vi "FLL Tournament Display Widescreen.vi"() -> ()   [LabVIEW 2013]
uses:
  Team_List_Ctrl.ctl
  Team_Scores_And_Rankings_Array_Ctrl.ctl
  Round_And_Score_Ctrl.ctl
  Timer_Details_Ctrl.ctl
  Sound Info.ctl
  <vilib>/sound2/lvsound2.llb/Sound Data Format.ctl
  <vilib>/sound2/lvsound2.llb/Sampling Mode.ctl
  SponsorImageFreqArray.ctl
  <vilib>/picture/picture.llb/imagedata.ctl
  <vilib>/sound2/lvsound2.llb/Sound Output Set Volume (Single).vi
  <vilib>/sound2/lvsound2.llb/Sound Output Write (DBL).vi
  <vilib>/httpClient/LabVIEWHTTPClient.lvlib
panel:
  out "TimerIP":string
  in  "Hurry-Up Sound Volume":dbl(slide)=88.46153846153847 scale=0.0..100.0
  in  "Pre-Match Coundown Sound Volume":dbl(slide)=88.46153846153847 scale=0.0..100.0
  in  "Uh-Oh Sound Volume":dbl(slide)=88.46153846153847 scale=0.0..100.0
  in  "Stop Sound Volume":dbl(slide)=100.0 scale=0.0..100.0
  in  "Start Sound Volume":dbl(slide)=100.0 scale=0.0..100.0
  out "Sound Cluster 2":T1={"Start"={"total number of samples/ch"=31680, "sound format"={"sample rate (S/s)"=11025.0, "number of channels"=1, "bits per sample"=16}, "data"=[{"t0"=timestamp(0 s since 1904-01-01), "dt"=9.070294784580499e-05, "Y"=array[31680 elements]}], "Volume"=100.0}, "Stop"={"total number of samples/ch"=27648, "sound format"={"sample rate (S/s)"=11025.0, "number of channels"=1, "bits per sample"=16}, "data"=[{"t0"=timestamp(0 s since 1904-01-01), "dt"=9.070294784580499e-05, "Y"=array[27648 elements]}], "Volume"=100.0}, "Uh-Oh"={"total number of samples/ch"=29952, "sound format"={"sample rate (S/s)"=11025.0, "number of channels"=1, "bits per sample"=16}, "data"=[{"t0"=timestamp(0 s since 1904-01-01), "dt"=9.070294784580499e-05, "Y"=array[29952 elements]}], "Volume"=88.46153846153847}, "PreMatch"={"total number of samples/ch"=225792, "sound format"={"sample rate (S/s)"=44100.0, "number of channels"=2, "bits per sample"=16}, "data"=[{"t0"=timestamp(0 s since 1904-01-01), "dt"=2.2675736961451248e-05, "Y"=array[225792 elements]}, {"t0"=timestamp(0 s since 1904-01-01), "dt"=2.2675736961451248e-05, "Y"=array[225792 elements]}], "Volume"=75.38461538461539}, "Hurry-Up"={"total number of samples/ch"=0, "sound format"={"sample rate (S/s)"=0.0, "number of channels"=0, "bits per sample"=0}, "data"=[], "Volume"=0.0}}
  in  "stop":bool
  in  "Sound To Play":T3(ring)
  out "Primary Sound Array":dbl[](array[numeric])
  out "PrePrimary Sound Array":dbl[](array[numeric])
  out "Secondary (s)":dbl
  out "Primary (s)":dbl
  out "Pre-Primary (s)":dbl
  out "Master Volume":dbl
  out "Sound Cluster":T1={"Start"={"total number of samples/ch"=31680, "sound format"={"sample rate (S/s)"=11025.0, "number of channels"=1, "bits per sample"=16}, "data"=[{"t0"=timestamp(0 s since 1904-01-01), "dt"=9.070294784580499e-05, "Y"=array[31680 elements]}], "Volume"=100.0}, "Stop"={"total number of samples/ch"=27648, "sound format"={"sample rate (S/s)"=11025.0, "number of channels"=1, "bits per sample"=16}, "data"=[{"t0"=timestamp(0 s since 1904-01-01), "dt"=9.070294784580499e-05, "Y"=array[27648 elements]}], "Volume"=100.0}, "Uh-Oh"={"total number of samples/ch"=29952, "sound format"={"sample rate (S/s)"=11025.0, "number of channels"=1, "bits per sample"=16}, "data"=[{"t0"=timestamp(0 s since 1904-01-01), "dt"=9.070294784580499e-05, "Y"=array[29952 elements]}], "Volume"=88.46153846153847}, "PreMatch"={"total number of samples/ch"=225792, "sound format"={"sample rate (S/s)"=44100.0, "number of channels"=2, "bits per sample"=16}, "data"=[{"t0"=timestamp(0 s since 1904-01-01), "dt"=2.2675736961451248e-05, "Y"=array[225792 elements]}, {"t0"=timestamp(0 s since 1904-01-01), "dt"=2.2675736961451248e-05, "Y"=array[225792 elements]}], "Volume"=75.38461538461539}, "Hurry-Up"={"total number of samples/ch"=0, "sound format"={"sample rate (S/s)"=0.0, "number of channels"=0, "bits per sample"=0}, "data"=[], "Volume"=0.0}}
  out "EnableSounds":bool
  out "Score Behavior":T4(ring)
  out "SFA":string[][](array[string])
  out "NumRoundsToShow":string
  out "Cancelled?":bool
  out "IP Address / Port":string
  in  "Scores Tab":enum32{"3 Rounds", "4 Rounds"}(tab)
  in  "Scores Box":i32[](listbox)
  in  "Scores Box 2":i32(listbox)=3
  in  "Top Tab":enum32{"Page 1"}(tab)
  out "Main Logo Image":picture
  out "Powered By LabVIEW":picture
  out "FIRST LEGO League":picture
  out "Match Indicator":string
  out "Tournament Title String":string="2013 FIRST LEGO League Nature's Fury"
  out "TIMER":string="2 : 3 0"
  out "Top Sponsor Image":picture
  out "Mid Sponsor Image":picture
  out "Bottom Sponsor Image":picture
  out "Timer Properties":T5
  out "Consolidated Scores and Rankings":T7(array[cluster])
  out "Reported Scores and Rankings":T8
  out "Full Team List":T9[](array[typedef])
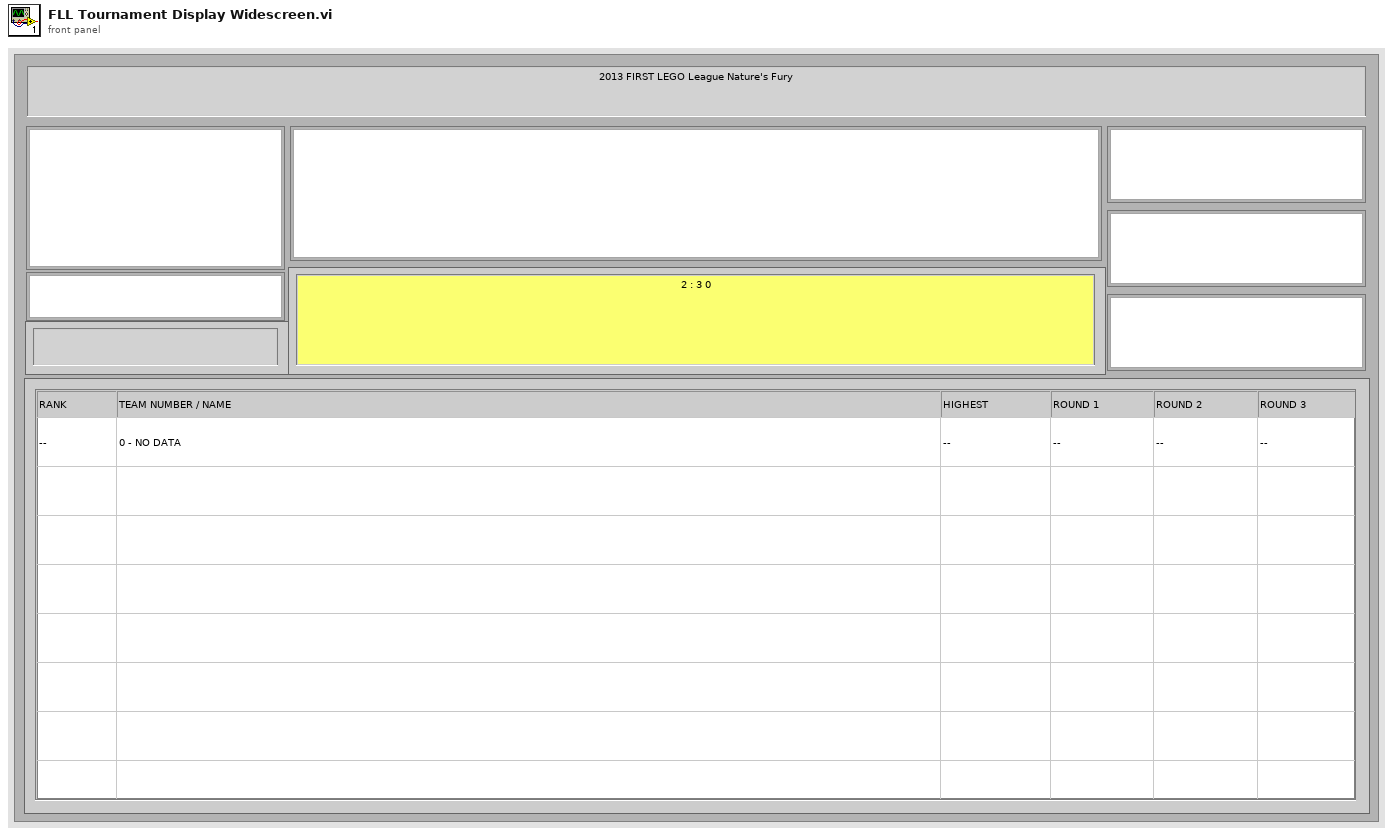
[diagram p1: front panel]
types:
  T1 = typedef "Sound Info.ctl" = cluster{"Start":cluster{"total number of samples/ch":u32, "sound format":T2, "data":waveform(dbl)[], "Volume":dbl}, "Stop":cluster{"total number of samples/ch":u32, "sound format":T2, "data":waveform(dbl)[], "Volume":dbl}, "Uh-Oh":cluster{"total number of samples/ch":u32, "sound format":T2, "data":waveform(dbl)[], "Volume":dbl}, "PreMatch":cluster{"total number of samples/ch":u32, "sound format":T2, "data":waveform(dbl)[], "Volume":dbl}, "Hurry-Up":cluster{"total number of samples/ch":u32, "sound format":T2, "data":waveform(dbl)[], "Volume":dbl}}
  T2 = typedef "Sound Data Format.ctl" = cluster{"sample rate (S/s)":dbl, "number of channels":i32, "bits per sample":i32}
  T3 = enum16{"None", "Start", "Stop", "Uh-Oh", "Prematch", "Hurry-Up"}
  T4 = enum16{"Show Negative Scores as ZERO", "Show Negative Scores"}
  T5 = typedef "Timer_Details_Ctrl.ctl" = cluster{"TimeRemaining":string, "MatchPhase":string, "CurrentMatch":string, "Timer_Running":string, "Seconds":string, "LastSound":string}
  T6 = typedef "Round_And_Score_Ctrl.ctl" = cluster{"Score":string, "Round Number":string}
  T7 = cluster{"Rank":string, "Team Number":string, "Team Name":string, "Highest Score":string, "Scores":T6[]}[]
  T8 = typedef "Team_Scores_And_Rankings_Array_Ctrl.ctl" = cluster{"Rank":string, "Team Number":string, "Team Name":string, "Highest Score":string, "Scores":T6[]}[]
  T9 = typedef "Team_List_Ctrl.ctl" = cluster{"Team Name":string, "Team Number":string}
  T10 = enum32{"Invalid", "Standard", "Closed", "Hidden", "Minimized", "Maximized"}
  T11 = cluster{"Master Volume":dbl, "Pre-Primary (s)":dbl, "Primary (s)":dbl, "Secondary (s)":dbl, "Start Sound Path":path, "Stop Sound Path":path, "Uh-Oh Sound Path":path, "Pre-Match Countdown Sound":path, "Hurry Up Sound":path, "Start Sound Volume":dbl, "Stop Sound Volume":dbl, "Uh-Oh Sound Volume":dbl, "Pre-Match Coundown Sound Volume":dbl, "Hurry Up Sound Volume":dbl}
  T12 = typedef "SponsorImageFreqArray.ctl" = cluster{"Cluster":cluster{"Array":T13[], "Frequency (s)":dbl}, "Cluster":cluster{"Array":T13[], "Frequency (s)":dbl}, "Cluster":cluster{"Array":T13[], "Frequency (s)":dbl}}
  T13 = typedef "imagedata.ctl" = cluster{"image type":i32, "image depth":i32, "image":u8[], "mask":u8[], "colors":u32[], "Rectangle":cluster{"left":i16, "top":i16, "right":i16, "bottom":i16}}
  T14 = typedef "LabVIEWHTTPClient.lvlib/ClientHandle.ctl" = refnum<k1>
  T15 = typedef "Team_List_Array_Ctrl.ctl" = T9[]
  T16 = cluster{"[0]":string, "[1]":string, "[2]":string, "[3]":string}
  T17 = enum32{"invalid app kind", "Development System", "Run Time System", "Student Edition", "Embedded LabVIEW", "Evaluation", "Custom"}
  T18 = cluster{"total number of samples/ch":u32, "sound format":T2, "data":waveform(dbl)[], "Volume":dbl}
  T19 = typedef "Sampling Mode.ctl" = i32
  T20 = typedef "Sound Output Task ID.ctl" = u32
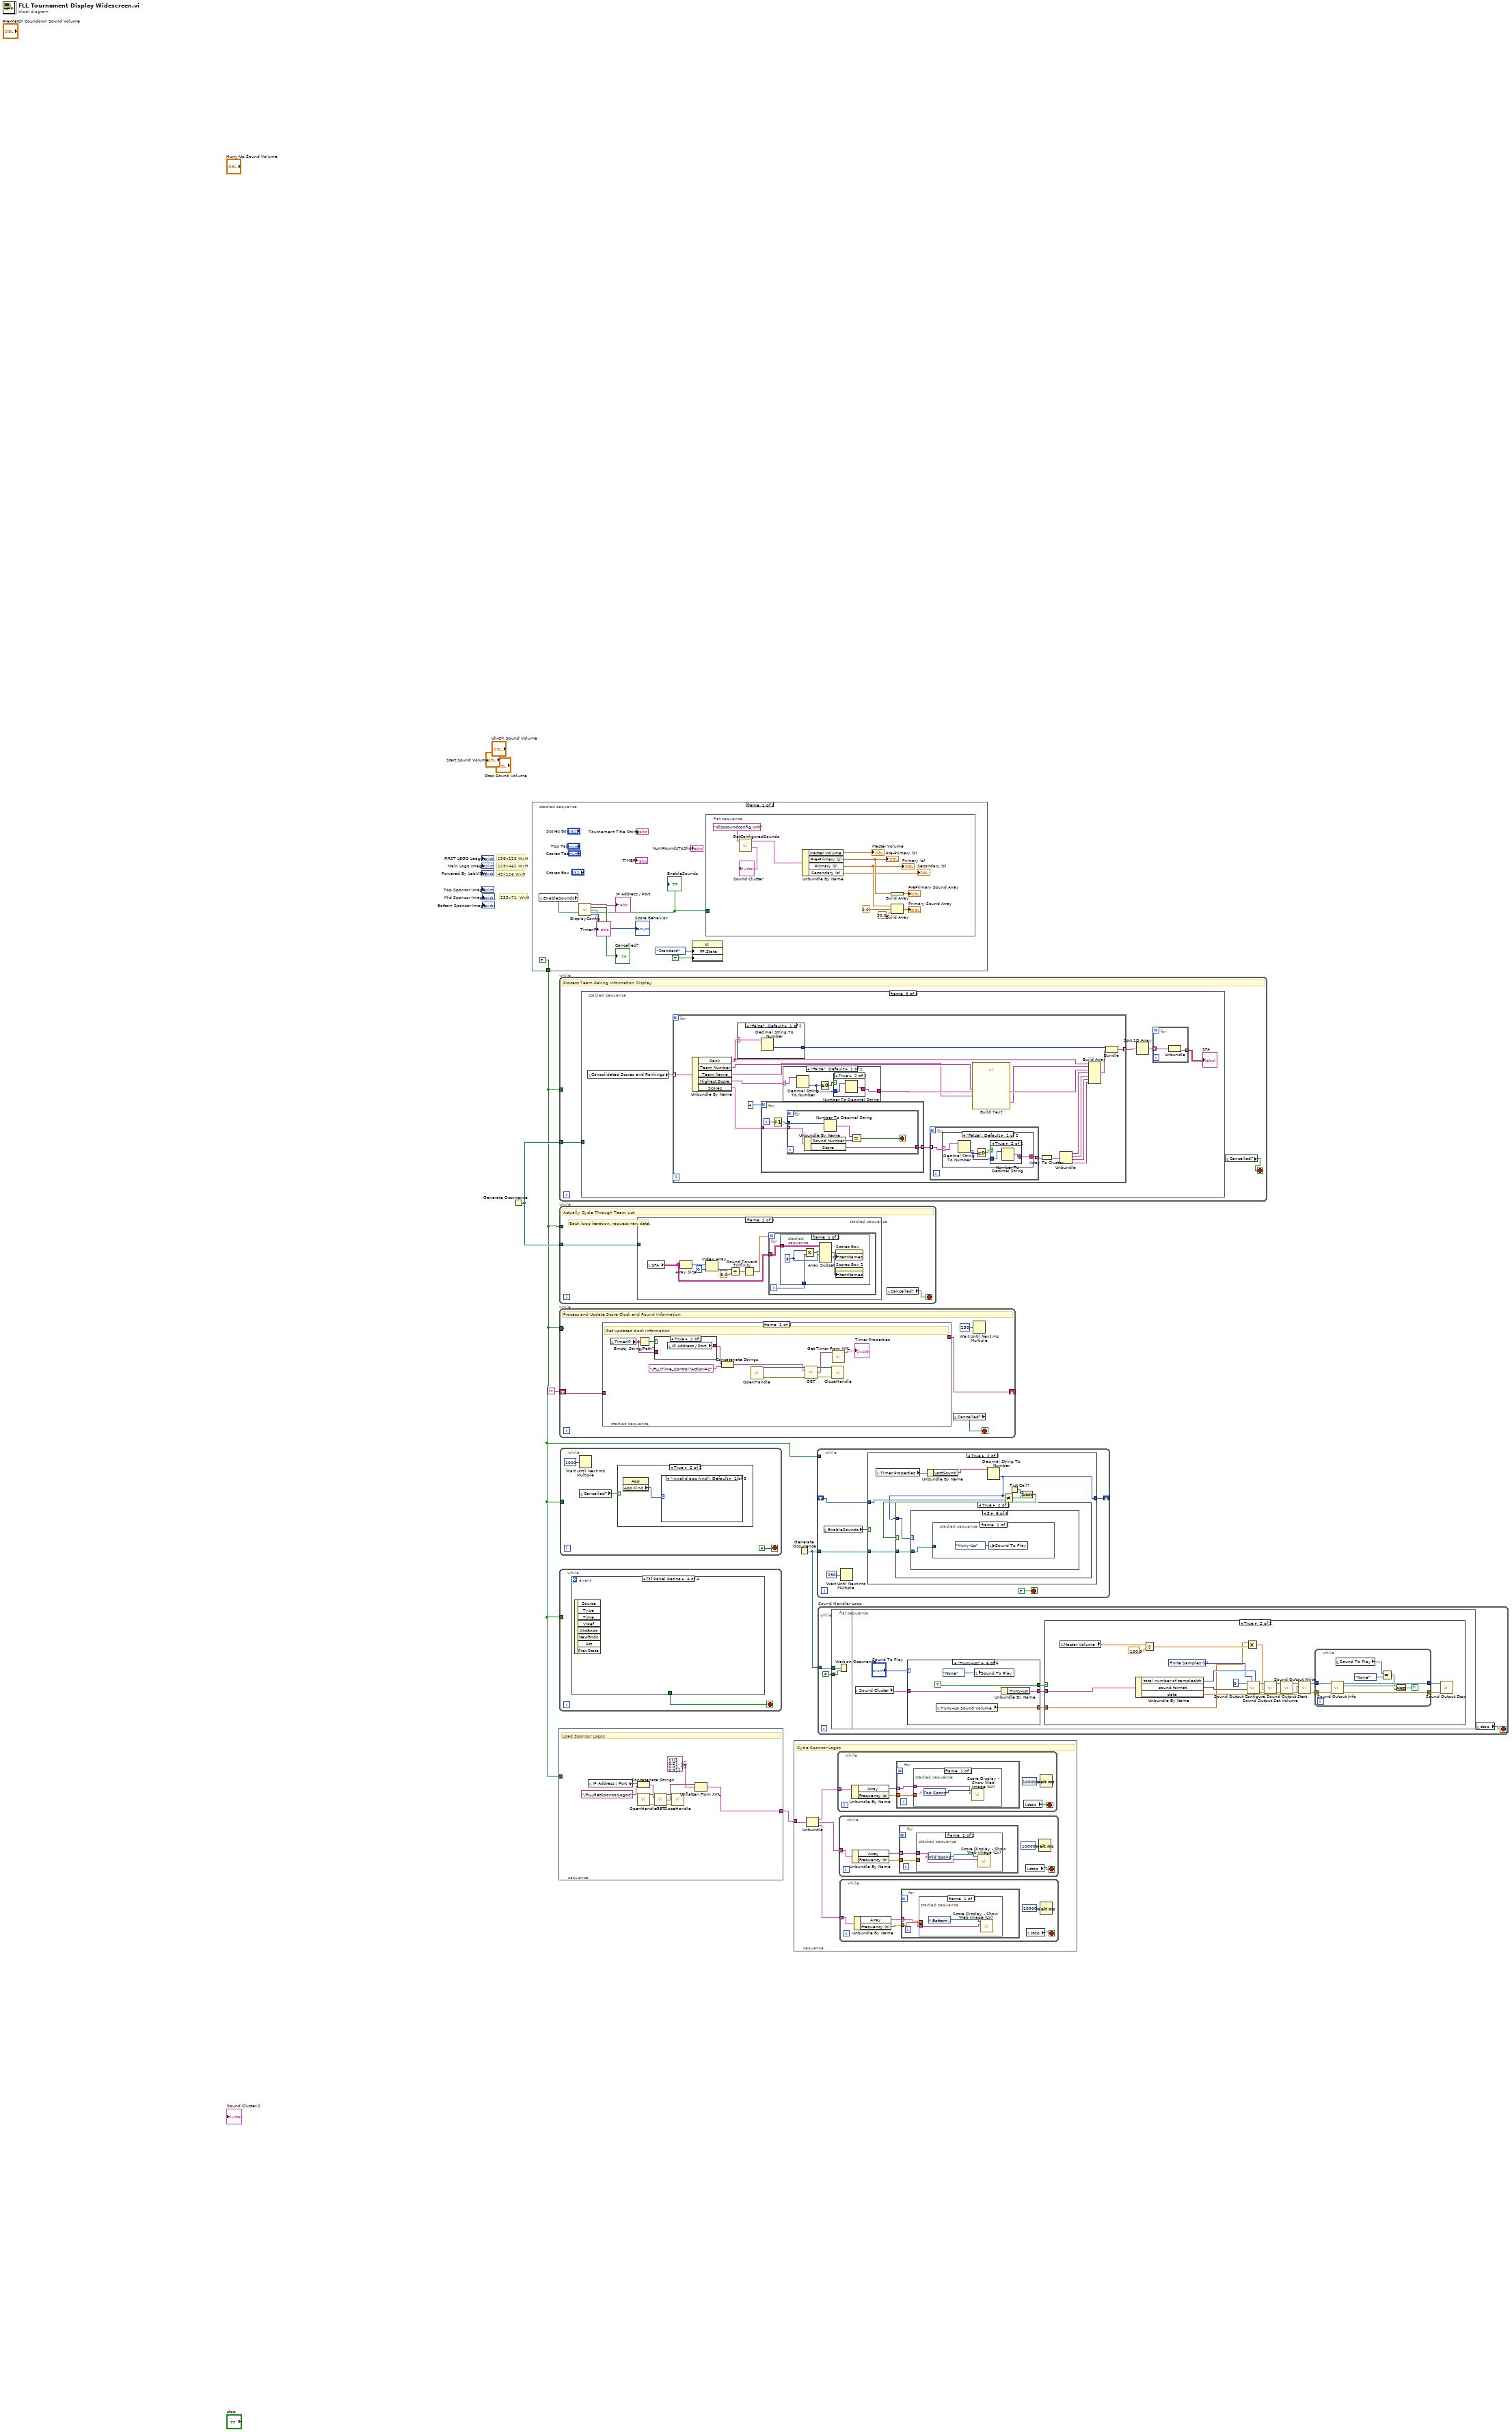
[diagram p0: block diagram]
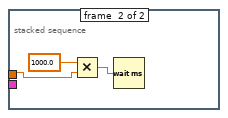
[diagram p2: hidden frame]
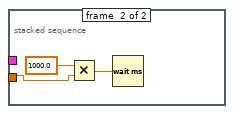
[diagram p3: hidden frame]
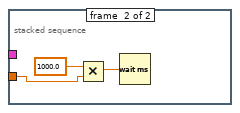
[diagram p4: hidden frame]
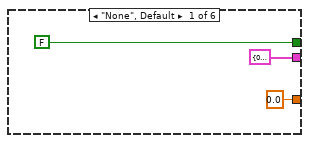
[diagram p6: hidden frame]
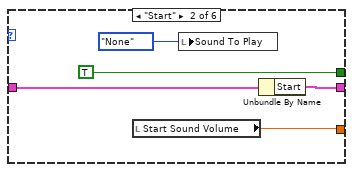
[diagram p7: hidden frame]
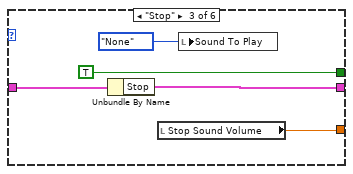
[diagram p8: hidden frame]
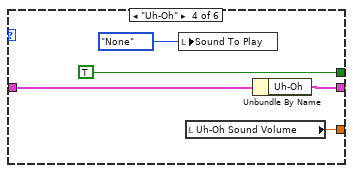
[diagram p9: hidden frame]
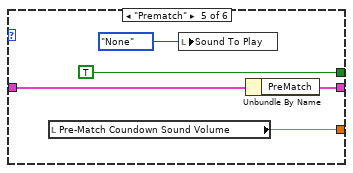
[diagram p10: hidden frame]
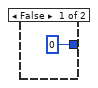
[diagram p11: hidden frame]
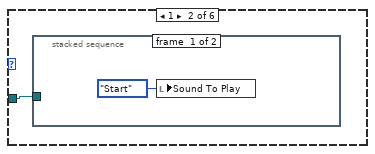
[diagram p14: hidden frame]
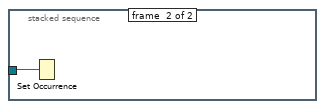
[diagram p15: hidden frame]
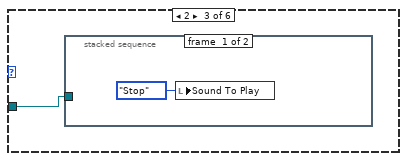
[diagram p16: hidden frame]
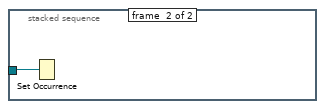
[diagram p17: hidden frame]
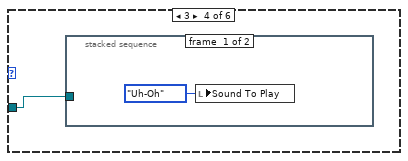
[diagram p18: hidden frame]
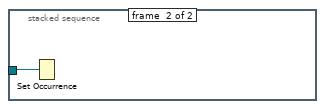
[diagram p19: hidden frame]
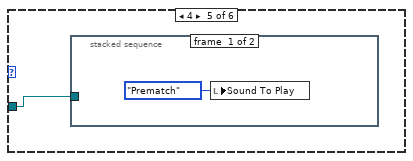
[diagram p20: hidden frame]
diagram:
  # "129x462 WxH"
  # "43x126 WxH"
  # "253x71  WxH"
  # "138x126 WxH"
  n1 = Generate Occurrence() -> (w4:refnum<k4>)
  n2 = stacked-sequence {
    tunnel: [FALSE _] -> w3
    frame #0 {
      n3 = local read "EnableSounds"() -> (w10:bool)
      n4 = call "DisplayConfig.vi"("EnableSounds"=w10) -> ("ScoreIP"=→"IP Address / Port":string, "Cancelled?"=→"Cancelled?":bool, "TimerIP"=→"TimerIP":string, "EnableSounds out"=w9:bool, "Score Behavior OUT"=→"Score Behavior":T4)  [unwired: 10 in]
      "EnableSounds" <- w9
      n5 = property class="VI"("FP.State"=T10."Standard" ("Front Panel Window:State"), "Front Panel.TitleBarVis"=TRUE ("Front Panel Window:Title Bar Visible")) -> ()  [unwired: 2 in, 2 out]
      n6 = flat-sequence {
        tunnel: w9 -> [_]
        frame #0 {
          n7 = call "GetConfiguredSounds.vi"("File"="dispsoundconfig.xml") -> ("Sound Cluster"=→"Sound Cluster":T1, "Settings Cluster"=w24:T11)  [unwired: 9 in]
          n8 = Unbundle By Name(w24) -> ("Master Volume"=→"Master Volume":dbl, "Pre-Primary (s)"=w21:dbl, "Primary (s)"=w19:dbl, "Secondary (s)"=→"Secondary (s)":dbl)
          "Pre-Primary (s)" <- w21
          "Primary (s)" <- w19
          n9 = Build Array(w21) -> (→"PrePrimary Sound Array":dbl[])
          n10 = Build Array(w19, 0.0 ("element"), 30.0 ("element")) -> (→"Primary Sound Array":dbl[])
        }
      }
    }
    frame #1 {
      n11 = disable-structure shown="Disabled" {
        frame Disabled {
          n12 = control-ref of="Powered By LabVIEW"() -> (w30:refnum<vi>)
          n13 = call "Score Display - Auto Scale Image (LV).vi"("Picture Reference"=w30, "path to image file"=path "C:/Users/Danny Diaz/Dropbox/FLL 2 (1).1/Images/powered-by-labview-horiz-logo-rgb.png") -> ()  [unwired: 1 out]
        }
        frame Enabled {
        }
      }
      n14 = disable-structure shown="Disabled" {
        frame Disabled {
          n15 = control-ref of="FIRST LEGO League"() -> (w28:refnum<vi>)
          n16 = call "Score Display - Auto Scale Image (LV).vi"("Picture Reference"=w28, "path to image file"=path "C:/Users/Danny Diaz/Dropbox/FLL 2 (1).1/Images/FLLicon_RGB.jpg") -> ()  [unwired: 1 out]
        }
        frame Enabled {
        }
      }
      n17 = disable-structure shown="Disabled" {
        frame Disabled {
          n18 = control-ref of="Main Logo Image"() -> (w26:refnum<vi>)
          n19 = call "Score Display - Auto Scale Image (LV).vi"("Picture Reference"=w26, "path to image file"=path "C:/Users/Danny Diaz/Dropbox/FLLTS2015/Images/TrashTrek_FNL.jpg") -> ()  [unwired: 1 out]
        }
        frame Enabled {
        }
      }
    }
  }
  n20 = stacked-sequence {
    tunnel: w3 -> [_]
    tunnel: [w32] -> w2
    frame #0 {
      # "Load Sponsor Logos"
      n21 = local read "IP Address / Port"() -> (w41:string)
      n22 = Concatenate Strings(w41, "/FLL/GetSponsorLogos" ("url")) -> (w40:string)
      n23 = call <vilib>:"OpenHandle.vi"() -> ("client handle out"=w36:T14, "error out"=w35:errorcluster)  [unwired: 14 in]
      n24 = call <vilib>:"GET.vi"("client handle"=w36, "url"=w40, "error in (no error)"=w35) -> ("client handle out"=w37:T14, "body"=w34:string, "error out"=w38:errorcluster)  [unwired: 9 in, 1 out]
      n25 = call <vilib>:"CloseHandle.vi"("client handle"=w37, "error in (no error)"=w38) -> ()  [unwired: 13 in, 1 out]
      n26 = Unflatten From XML(xml string=w34, type=T12 {"Cluster"={"Array"=[], "Frequency (s)"=0.0}, "Cluster"={"Array"=[], "Frequency (s)"=0.0}, "Cluster"={"Array"=[], "Frequency (s)"=0.0}} ("output cluster")) -> (value=w32:T12)  [unwired: 1 in, 1 out]
    }
  }
  n27 = while {
    tunnel: w3 -> [_]
    tunnel: w4 -> [w42]
    stop <- w43 stop-if-true
    # "Process Team Raking Information Display"
    n28 = stacked-sequence {
      tunnel: w42 -> [w44 _ _ _]
      frame #0 {
        # "Wait for request before acquiring new set of data."
        n29 = Wait on Occurrence(2:w44) -> ()  [unwired: 2 in, 1 out]
      }
      frame #1 {
        # "Get Teams and Scores, and Consolidate into a unified team view"
        n30 = local read "IP Address / Port"() -> (w47:string)
        n31 = Concatenate Strings(w47, "/FLL/Get_Num_Rounds_To_Show" ("url")) -> (w46:string)
        n32 = Concatenate Strings(w47, "/FLL/Serve_Team_Data" ("url")) -> (w61:string)
        n33 = Concatenate Strings(w47, "/FLL/Get_Team_Ranking_Web" ("url")) -> (w59:string)
        n34 = Concatenate Strings(w47, "/FLL/Get_Game_Title" ("url")) -> (w54:string)
        n35 = call <vilib>:"OpenHandle.vi"() -> ("client handle out"=w70:T14, "error out"=w68:errorcluster)  [unwired: 14 in]
        n36 = call <vilib>:"GET.vi"("client handle"=w70, "url"=w59, "error in (no error)"=w68) -> ("client handle out"=w67:T14, "body"=w66:string, "error out"=w69:errorcluster)  [unwired: 9 in, 1 out]
        n37 = call "Get Scores from XML.vi"("XML In"=w66) -> ("Team_Scores_And_Rankings_Array"=w64:T7)  [unwired: 10 in]
        "Reported Scores and Rankings" <- w64
        n38 = call <vilib>:"GET.vi"("client handle"=w67, "url"=w61, "error in (no error)"=w69) -> ("client handle out"=w58:T14, "body"=w56:string, "error out"=w57:errorcluster)  [unwired: 9 in, 1 out]
        n39 = call <vilib>:"GET.vi"("client handle"=w58, "url"=w54, "error in (no error)"=w57) -> ("client handle out"=w49:T14, "body"=w53:string, "error out"=w50:errorcluster)  [unwired: 9 in, 1 out]
        n40 = call <vilib>:"GET.vi"("client handle"=w49, "url"=w46, "error in (no error)"=w50) -> ("client handle out"=w52:T14, "body"=w45:string, "error out"=w51:errorcluster)  [unwired: 9 in, 1 out]
        n41 = local write "NumRoundsToShow"(w45) -> ()
        n42 = call <vilib>:"CloseHandle.vi"("client handle"=w52, "error in (no error)"=w51) -> ()  [unwired: 13 in, 1 out]
        n43 = local write "Tournament Title String"(w53) -> ()
        n44 = call "Get Team List from XML.vi"("XML In"=w56) -> ("Team List Array"=w65:T15)  [unwired: 10 in]
        "Full Team List" <- w65
        n45 = call "Consolidate Teams and Rankings.vi"("Team List Array"=w65, "Team_Scores_And_Rankings_Array"=w64) -> ("Consolidated Teams and Rankings"=→"Consolidated Scores and Rankings":T7)  [unwired: 9 in]
      }
      frame #2 {
        n46 = local read "Consolidated Scores and Rankings"() -> (w74:T7)
        n47 = for {
          tunnel: w74 -> [w85] mode=indexing
          tunnel: [w84] -> w72 mode=indexing
          n48 = Unbundle By Name(w85) -> ("Rank"=w87:string, "Team Number"=w79:string, "Team Name"=w78:string, "Highest Score"=w83:string, "Scores"=w95:T6[])
          n49 = case shown="\"False\", Default" w87 {
            selector: w87 -> [w115 _]
            tunnel: [w114 1000] -> w86
            frame "False", Default {
              n50 = Decimal String To Number(string=w115) -> (number=w114:i32)  [unwired: 2 in, 1 out]
            }
            frame "--" {
            }
          }
          n51 = for {
            N: 4 -> [_]
            tunnel: w95 -> [w119]
            tunnel: [w117] -> w81 mode=indexing
            i -> [w120]
            n52 = Increment(x=w120) -> (x+1=w118:i32)
            n53 = for {
              tunnel: w119 -> [w122] mode=indexing
              tunnel: w118 -> [w126]
              tunnel: [w121] -> w117
              stop <- w123 stop-if-true
              n54 = Unbundle By Name(w122) -> ("Round Number"=w125:string, "Score"=w121:string)
              n55 = Number To Decimal String(number=w126) -> (decimal integer string=w124:string)  [unwired: 1 in]
              n56 = Equal?(x=w124, y=w125) -> (x = y?=w123:bool)
            }
          }
          n57 = case shown="\"False\", Default" w83 {
            selector: w83 -> [w109 w113]
            tunnel: [w107 w113] -> w82
            frame "False", Default {
              n58 = Decimal String To Number(string=w109) -> (number=w106:i32)  [unwired: 2 in, 1 out]
              n59 = Greater Or Equal To 0?(x=w106) -> (x >= 0?=w108:bool)
              n60 = case shown="True" w108 {
                tunnel: ["0" w112] -> w107
                tunnel: w106 -> [_ w111]
                frame False {
                }
                frame True {
                  n61 = Number To Decimal String(number=w111) -> (decimal integer string=w112:string)  [unwired: 1 in]
                }
              }
            }
            frame "--" {
            }
          }
          n62 = for {
            tunnel: w81 -> [w97] mode=indexing
            tunnel: [w96] -> w80 mode=indexing
            n63 = case shown="\"False\", Default" w97 {
              selector: w97 -> [w100 w105]
              tunnel: [w101 w105] -> w96
              frame "False", Default {
                n64 = Decimal String To Number(string=w100) -> (number=w98:i32)  [unwired: 2 in, 1 out]
                n65 = Greater Or Equal To 0?(x=w98) -> (x >= 0?=w99:bool)
                n66 = case shown="True" w99 {
                  tunnel: ["0" w104] -> w101
                  tunnel: w98 -> [_ w103]
                  frame False {
                  }
                  frame True {
                    n67 = Number To Decimal String(number=w103) -> (decimal integer string=w104:string)  [unwired: 1 in]
                  }
                }
              }
              frame "--" {
              }
            }
          }
          n68 = call "Build Text"("team_number"=w79, "team_name"=w78) -> ("Result"=w77:string)  [unwired: 12 in, 1 out]
          n69 = Array To Cluster(array=w80) -> (cluster=w93:T16)
          n70 = Unbundle(w93) -> ("[0]"=w92:string, "[1]"=w91:string, "[2]"=w90:string, "[3]"=w89:string)
          n71 = Build Array(w87, w77, w82, w92, w91, w90, w89) -> (w88:string[])
          n72 = Bundle(w86, w88) -> (w84:cluster{i32, string[]})  [unwired: 1 in]
        }
        n73 = Sort 1D Array(array=w72) -> (sorted array=w73:cluster{i32, string[]}[])
        n74 = for {
          tunnel: w73 -> [w76] mode=indexing
          tunnel: [w75] -> w71 mode=indexing
          n75 = Unbundle(w76) -> (w75:string[])  [unwired: 1 out]
        }
        "SFA" <- w71
      }
      frame #3 {
        n76 = local read "NumRoundsToShow"() -> (w127:string)
        n77 = case shown="\"1\"" w127 {
          frame "0", Default {
            n78 = local write "Scores Tab"(enum32{"3 Rounds", "4 Rounds"}."3 Rounds" ("Scores Tab")) -> ()
          }
          frame "1" {
            n79 = local write "Scores Tab"(enum32{"3 Rounds", "4 Rounds"}."4 Rounds" ("Scores Tab")) -> ()
          }
        }
      }
    }
    n80 = local read "Cancelled?"() -> (w43:bool)
  }
  n81 = while {
    tunnel: w3 -> [_]
    tunnel: w4 -> [w130]
    stop <- w131 stop-if-true
    # "Each loop iteration, request new data."
    # "Actually Cycle Through Team List"
    n82 = stacked-sequence {
      tunnel: w130 -> [w132 _ _]
      frame #0 {
        n83 = Set Occurrence(w132) -> ()
      }
      frame #1 {
        n84 = local read "SFA"() -> (w133:string[][])
        n85 = Array Size(array=w133) -> (size(s)=w138:i32[])
        n86 = Index Array(array=w138, index=0) -> (element=w139:i32)
        n87 = Divide(x=w139, y=8.0) -> (x/y=w135:dbl)
        n88 = Round Toward +Infinity(x=w135) -> (ceil(x): smallest int >= x=w136:dbl)
        n89 = for {
          N: w136 -> [_]
          tunnel: w133 -> [w141]
          i -> [w140]
          n90 = stacked-sequence {
            tunnel: w141 -> [w146 _]
            tunnel: w140 -> [w145 _]
            frame #0 {
              w144 = 8 ("length")
              n91 = Multiply(x=w144, y=w145) -> (x*y=w143:i32)
              n92 = Array Subset(array=w146, index (row)=w143, length (row)=w144) -> (w142:string[][])  [unwired: 2 in]
              n93 = property on="Scores Box" class="MCListbox (strict)"("ItemNames"=w142) -> ()  [unwired: 2 in, 2 out]
              n94 = property on="Scores Box 2" class="MCListbox (strict)"("ItemNames"=w142) -> ()  [unwired: 2 in, 2 out]
            }
            frame #1 {
              n95 = Wait Until Next ms Multiple(millisecond multiple=u32 6000) -> ()  [unwired: 1 out]
            }
          }
        }
      }
      frame #2 {
        n96 = Wait Until Next ms Multiple(millisecond multiple=u32 500) -> ()  [unwired: 1 out]
      }
    }
    n97 = local read "Cancelled?"() -> (w131:bool)
  }
  n98 = while {
    shift-right: [w151] -> _
    shift-left: "" -> [w152]
    tunnel: [w150] -> _
    tunnel: w3 -> [w150]
    stop <- w149 stop-if-true
    # "Process and Update Score Clock and Round Information"
    n99 = stacked-sequence {
      tunnel: w152 -> [_ w170 _]
      tunnel: [_ w169 _] -> w151
      frame #0 {
        # "Get updated clock information"
        n100 = local read "TimerIP"() -> (w154:string)
        n101 = Empty String/Path?(string/path=w154) -> (empty?=w155:bool)
        n102 = case shown="True" w155 {
          tunnel: [w165 w166] -> w158
          tunnel: w154 -> [w165 _]
          frame False {
          }
          frame True {
            n103 = local read "IP Address / Port"() -> (w166:string)
          }
        }
        n104 = Concatenate Strings(w158, "/FLL/Time_Control?Action=2" ("url")) -> (w156:string)
        n105 = call <vilib>:"OpenHandle.vi"() -> ("client handle out"=w163:T14, "error out"=w161:errorcluster)  [unwired: 14 in]
        n106 = call <vilib>:"GET.vi"("client handle"=w163, "url"=w156, "error in (no error)"=w161) -> ("client handle out"=w162:T14, "body"=w159:string, "error out"=w160:errorcluster)  [unwired: 9 in, 1 out]
        n107 = call <vilib>:"CloseHandle.vi"("client handle"=w162, "error in (no error)"=w160) -> ()  [unwired: 13 in, 1 out]
        n108 = call "Get Timer From XML.vi"("body"=w159) -> ("Cluster"=→"Timer Properties":T5)  [unwired: 9 in, 1 out]
      }
      frame #1 {
        n109 = local read "Timer Properties"() -> (w172:T5)
        n110 = local read "Timer Properties"() -> (w168:T5)
        n111 = Unbundle By Name(w172) -> ("TimeRemaining"=w169:string)
        n112 = Unbundle By Name(w168) -> ("MatchPhase"=w167:string)
        n113 = Equal?(x=w169, y=w170) -> (x = y?=w171:bool)
        n114 = case shown="True" w171 {
          tunnel: w169 -> [_ w175]
          tunnel: w167 -> [_ w173]
          frame False {
          }
          frame True {
            n115 = case shown="\"2\"" w173 {
              tunnel: [u32 16514929 u32 11272072 u32 16746633 u32 16774656] -> w174
              frame "3", Default {
              }
              frame "1" {
              }
              frame "2" {
              }
              frame "0" {
              }
            }
            n116 = property on="TIMER" class="Str"("Text.BGColor"=w174) -> ()  [unwired: 2 in, 2 out]
            n117 = local write "TIMER"(w175) -> ()
          }
        }
      }
      frame #2 {
        n118 = local read "Timer Properties"() -> (w184:T5)
        n119 = Unbundle By Name(w184) -> ("CurrentMatch"=w182:string)
        n120 = Concatenate Strings("MATCH", " " ("string"), w182) -> (→"Match Indicator":string)
      }
    }
    n121 = local read "Cancelled?"() -> (w149:bool)
    n122 = Wait Until Next ms Multiple(millisecond multiple=u32 250) -> ()  [unwired: 1 out]
  }
  n123 = while {
    tunnel: w3 -> [_]
    stop <- w185 stop-if-true
    n124 = event shown="[3] Panel Resize" {
      selector: _ -> [_ _ _ _]
      dyn-events: _ -> [_ _ _ _]
      timeout: _ -> [_ _ _ _]
      tunnel: [FALSE _ FALSE _] -> w185
      event Timeout {
        n125 = event-data() -> ()  [unwired: 1 in, 2 out]
      }
      event Key Down {
        n126 = event-data() -> ("Char"=w188:i16, "ScanCode"=w187:i16)  [unwired: 1 in, 7 out]
        n127 = case shown="32" w188 {
          tunnel: w187 -> [_ w200 _]
          frame 32 {
            n128 = property class="VI"() -> ("FP.State"=w189:T10)  [unwired: 2 in, 2 out]
            n129 = case shown="\"Standard\"" w189 {
              frame "Invalid", Default {
              }
              frame "Standard" {
                n130 = property class="VI"("FP.State"=T10."Maximized" ("Front Panel Window:State"), "Front Panel.TitleBarVis"=FALSE ("Front Panel Window:Title Bar Visible")) -> ()  [unwired: 2 in, 2 out]
              }
              frame "Closed" {
                n131 = property class="VI"("FP.State"=T10."Standard" ("Front Panel Window:State"), "Front Panel.TitleBarVis"=TRUE ("Front Panel Window:Title Bar Visible")) -> ()  [unwired: 2 in, 2 out]
              }
              frame "Hidden" {
                n132 = property class="VI"("FP.State"=T10."Standard" ("Front Panel Window:State"), "Front Panel.TitleBarVis"=TRUE ("Front Panel Window:Title Bar Visible")) -> ()  [unwired: 2 in, 2 out]
              }
              frame "Minimized" {
                n133 = property class="VI"("FP.State"=T10."Standard" ("Front Panel Window:State"), "Front Panel.TitleBarVis"=TRUE ("Front Panel Window:Title Bar Visible")) -> ()  [unwired: 2 in, 2 out]
              }
              frame "Maximized" {
                n134 = property class="VI"("FP.State"=T10."Standard" ("Front Panel Window:State"), "Front Panel.TitleBarVis"=TRUE ("Front Panel Window:Title Bar Visible")) -> ()  [unwired: 2 in, 2 out]
              }
            }
          }
          frame 1, Default {
            n135 = case shown="1" w200 {
              frame 0, Default {
              }
              frame 1 {
                n136 = local read "EnableSounds"() -> (w203:bool)
                n137 = call "DisplayConfig.vi"("EnableSounds"=w203) -> ("ScoreIP"=w205:string, "Cancelled?"=w206:bool, "TimerIP"=w201:string, "EnableSounds out"=w202:bool, "Score Behavior OUT"=w204:T4)  [unwired: 10 in]
                n138 = local write "IP Address / Port"(w205) -> ()
                n139 = local write "Score Behavior"(w204) -> ()
                n140 = local write "EnableSounds"(w202) -> ()
                n141 = local write "Cancelled?"(w206) -> ()
                n142 = local write "TimerIP"(w201) -> ()
              }
            }
          }
          frame 27 {
            # "Pressed C"
          }
        }
      }
      event Panel Close? {
        n143 = event-data() -> ()  [unwired: 1 in, 4 out]
        n144 = local read "EnableSounds"() -> (w209:bool)
        n145 = call "DisplayConfig.vi"("EnableSounds"=w209) -> ("ScoreIP"=w214:string, "Cancelled?"=w212:bool, "TimerIP"=w207:string, "EnableSounds out"=w208:bool, "Score Behavior OUT"=w210:T4)  [unwired: 10 in]
        n146 = local write "IP Address / Port"(w214) -> ()
        n147 = local write "Score Behavior"(w210) -> ()
        n148 = local write "EnableSounds"(w208) -> ()
        n149 = local write "Cancelled?"(w212) -> ()
        n150 = local write "TimerIP"(w207) -> ()
        n151 = Not(x=w212) -> (.not. x?=w213:bool)
        n152 = event-data("Discard?"=w213) -> ()  [unwired: 1 in, 1 out]
      }
      event Panel Resize {
        n153 = event-data() -> ()  [unwired: 1 in, 8 out]
      }
    }
  }
  n154 = while {
    tunnel: w3 -> [_]
    stop <- FALSE stop-if-true
    n155 = Wait Until Next ms Multiple(millisecond multiple=u32 1000) -> ()  [unwired: 1 out]
    n156 = local read "Cancelled?"() -> (w217:bool)
    n157 = case shown="True" w217 {
      frame False {
      }
      frame True {
        n158 = property class="App"() -> ("App.Kind"=w218:T17)  [unwired: 2 in, 2 out]
        n159 = case shown="\"invalid app kind\", Default" w218 {
          frame "invalid app kind", Default {
          }
          frame "Development System" {
            n160 = Stop(stop? (T)=TRUE) -> ()
          }
          frame "Run Time System" {
            n161 = Quit LabVIEW(quit? (T)=TRUE ("stop? (T)")) -> ()
          }
        }
      }
    }
  }
  n162 = stacked-sequence {
    tunnel: w2 -> [w224]
    frame #0 {
      # "Cycle Sponsor Logos"
      n163 = Unbundle(w224) -> ("Cluster"=w223:cluster{"Array":T13[], "Frequency (s)":dbl}, "Cluster"=w222:cluster{"Array":T13[], "Frequency (s)":dbl}, "Cluster"=w221:cluster{"Array":T13[], "Frequency (s)":dbl})
      n164 = while {
        tunnel: w223 -> [w252]
        stop <- w253 stop-if-true
        n165 = Unbundle By Name(w252) -> ("Array"=w251:T13[], "Frequency (s)"=w250:dbl)
        n166 = for {
          tunnel: w251 -> [w254] mode=indexing
          tunnel: w250 -> [w255]
          n167 = stacked-sequence {
            tunnel: w255 -> [_ w258]
            tunnel: w254 -> [w256 _]
            frame #0 {
              n168 = control-ref of="Top Sponsor Image"() -> (w257:refnum<vi>)
              n169 = call "Score Display - Show Web Image (LV).vi"("image data"=w256, "Picture in"=w257) -> ()  [unwired: 10 in]
            }
            frame #1 {
              n170 = Multiply(x=1000.0, y=w258) -> (x*y=w259:dbl)
              n171 = Wait (ms)(milliseconds to wait=w259) -> ()  [unwired: 1 out]
            }
          }
        }
        n172 = local read "stop"() -> (w253:bool)
        n173 = Wait (ms)(milliseconds to wait=u32 10000) -> ()  [unwired: 1 out]
      }
      n174 = while {
        tunnel: w222 -> [w240]
        stop <- w241 stop-if-true
        n175 = Unbundle By Name(w240) -> ("Array"=w239:T13[], "Frequency (s)"=w238:dbl)
        n176 = for {
          tunnel: w239 -> [w242] mode=indexing
          tunnel: w238 -> [w243]
          n177 = stacked-sequence {
            tunnel: w243 -> [_ w246]
            tunnel: w242 -> [w244 _]
            frame #0 {
              n178 = control-ref of="Mid Sponsor Image"() -> (w245:refnum<vi>)
              n179 = call "Score Display - Show Web Image (LV).vi"("image data"=w244, "Picture in"=w245) -> ()  [unwired: 10 in]
            }
            frame #1 {
              n180 = Multiply(x=1000.0, y=w246) -> (x*y=w247:dbl)
              n181 = Wait (ms)(milliseconds to wait=w247) -> ()  [unwired: 1 out]
            }
          }
        }
        n182 = local read "stop"() -> (w241:bool)
        n183 = Wait (ms)(milliseconds to wait=u32 10000) -> ()  [unwired: 1 out]
      }
      n184 = while {
        tunnel: w221 -> [w228]
        stop <- w229 stop-if-true
        n185 = Unbundle By Name(w228) -> ("Array"=w227:T13[], "Frequency (s)"=w226:dbl)
        n186 = for {
          tunnel: w227 -> [w230] mode=indexing
          tunnel: w226 -> [w231]
          n187 = stacked-sequence {
            tunnel: w231 -> [_ w234]
            tunnel: w230 -> [w232 _]
            frame #0 {
              n188 = control-ref of="Bottom Sponsor Image"() -> (w233:refnum<vi>)
              n189 = call "Score Display - Show Web Image (LV).vi"("image data"=w232, "Picture in"=w233) -> ()  [unwired: 10 in]
            }
            frame #1 {
              n190 = Multiply(x=1000.0, y=w234) -> (x*y=w235:dbl)
              n191 = Wait (ms)(milliseconds to wait=w235) -> ()  [unwired: 1 out]
            }
          }
        }
        n192 = local read "stop"() -> (w229:bool)
        n193 = Wait (ms)(milliseconds to wait=u32 10000) -> ()  [unwired: 1 out]
      }
    }
  }
  n194 = Generate Occurrence() -> (w1:refnum<k4>)
  n195 = while {
    tunnel: w3 -> [_]
    shift-right: [w263] -> _
    shift-left: _ -> [w262]
    tunnel: w1 -> [w261]
    stop <- FALSE stop-if-true
    n196 = local read "EnableSounds"() -> (w264:bool)
    n197 = Wait Until Next ms Multiple(millisecond multiple=u32 250) -> ()  [unwired: 1 out]
    n198 = case shown="True" w264 {
      tunnel: [0 w271] -> w263
      tunnel: w262 -> [_ w275]
      tunnel: w261 -> [_ w268]
      frame False {
      }
      frame True {
        n199 = local read "Timer Properties"() -> (w270:T5)
        n200 = Unbundle By Name(w270) -> ("LastSound"=w269:string)
        n201 = Decimal String To Number(string=w269) -> (number=w271:i32)  [unwired: 2 in, 1 out]
        n202 = Not Equal?(x=w271, y=w275) -> (x != y?=w273:bool)
        n203 = First Call?() -> (First Call?: T/F=w274:bool)
        n204 = Compound Arithmetic op=AND(invert w274, w273) -> (w272:bool)
        n205 = case shown="True" w272 {
          tunnel: w271 -> [_ w277]
          tunnel: w268 -> [_ w276]
          frame False {
          }
          frame True {
            n206 = case shown="5" w277 {
              tunnel: w276 -> [_ w278 w281 w284 w287 w290]
              frame 0, Default {
              }
              frame 1 {
                n207 = stacked-sequence {
                  tunnel: w278 -> [_ w280]
                  frame #0 {
                    n208 = local write "Sound To Play"(T3."Start" ("Sound To Play")) -> ()
                  }
                  frame #1 {
                    n209 = Set Occurrence(w280) -> ()
                  }
                }
              }
              frame 2 {
                n210 = stacked-sequence {
                  tunnel: w281 -> [_ w283]
                  frame #0 {
                    n211 = local write "Sound To Play"(T3."Stop" ("Sound To Play")) -> ()
                  }
                  frame #1 {
                    n212 = Set Occurrence(w283) -> ()
                  }
                }
              }
              frame 3 {
                n213 = stacked-sequence {
                  tunnel: w284 -> [_ w286]
                  frame #0 {
                    n214 = local write "Sound To Play"(T3."Uh-Oh" ("Sound To Play")) -> ()
                  }
                  frame #1 {
                    n215 = Set Occurrence(w286) -> ()
                  }
                }
              }
              frame 4 {
                n216 = stacked-sequence {
                  tunnel: w287 -> [_ w289]
                  frame #0 {
                    n217 = local write "Sound To Play"(T3."Prematch" ("Sound To Play")) -> ()
                  }
                  frame #1 {
                    n218 = Set Occurrence(w289) -> ()
                  }
                }
              }
              frame 5 {
                n219 = stacked-sequence {
                  tunnel: w290 -> [_ w292]
                  frame #0 {
                    n220 = local write "Sound To Play"(T3."Hurry-Up" ("Sound To Play")) -> ()
                  }
                  frame #1 {
                    n221 = Set Occurrence(w292) -> ()
                  }
                }
              }
            }
          }
        }
      }
    }
  }
  n222 = while "Sound Handler Loop" {
    tunnel: w1 -> [w294]
    stop <- w295 stop-if-true
    n223 = flat-sequence {
      tunnel: w294 -> [w297]
      tunnel: FALSE ("ignore previous (T)") -> [w296]
      frame #0 {
        n224 = Wait on Occurrence(1:w296, 2:w297) -> ()  [unwired: 1 in, 1 out]
      }
      frame #1 {
        n225 = local read "Sound Cluster"() -> (w301:T1)
        n226 = case shown="\"Hurry-Up\"" "Sound To Play" {
          tunnel: w301 -> [_ w340 w345 w350 w355 w360]
          tunnel: [T18 {"total number of samples/ch"=0, "sound format"={"sample rate (S/s)"=0.0, "number of channels"=0, "bits per sample"=0}, "data"=[], "Volume"=0.0} ("Uh-Oh") w339 w344 w348 w353 w358] -> w300
          tunnel: [FALSE TRUE TRUE TRUE TRUE TRUE] -> w299
          tunnel: [0.0 ("Pre-Match Coundown Sound Volume") w336 w341 w346 w351 w356] -> w298
          frame "None", Default {
          }
          frame "Start" {
            n227 = local read "Start Sound Volume"() -> (w336:dbl)
            n228 = local write "Sound To Play"(enum16{"None", "Start", "Stop", "Uh-Oh"}."None" ("Sound To Play")) -> ()
            n229 = Unbundle By Name(w340) -> ("Start"=w339:T18)
          }
          frame "Stop" {
            n230 = Unbundle By Name(w345) -> ("Stop"=w344:T18)
            n231 = local read "Stop Sound Volume"() -> (w341:dbl)
            n232 = local write "Sound To Play"(enum16{"None", "Start", "Stop", "Uh-Oh"}."None" ("Sound To Play")) -> ()
          }
          frame "Uh-Oh" {
            n233 = local write "Sound To Play"(enum16{"None", "Start", "Stop", "Uh-Oh"}."None" ("Sound To Play")) -> ()
            n234 = local read "Uh-Oh Sound Volume"() -> (w346:dbl)
            n235 = Unbundle By Name(w350) -> ("Uh-Oh"=w348:T18)
          }
          frame "Prematch" {
            n236 = local read "Pre-Match Coundown Sound Volume"() -> (w351:dbl)
            n237 = local write "Sound To Play"(enum16{"None", "Start", "Stop", "Uh-Oh"}."None" ("Sound To Play")) -> ()
            n238 = Unbundle By Name(w355) -> ("PreMatch"=w353:T18)
          }
          frame "Hurry-Up" {
            n239 = local read "Hurry-Up Sound Volume"() -> (w356:dbl)
            n240 = local write "Sound To Play"(enum16{"None", "Start", "Stop", "Uh-Oh"}."None" ("Sound To Play")) -> ()
            n241 = Unbundle By Name(w360) -> ("Hurry-Up"=w358:T18)
          }
        }
        n242 = case shown="True" w299 {
          tunnel: w300 -> [_ w323]
          tunnel: w298 -> [_ w304]
          frame False {
          }
          frame True {
            w321 = T19 0 items=["Finite Samples", "Continuous Samples"] ("sample mode")
            n243 = local read "Master Volume"() -> (w303:dbl)
            n244 = Unbundle By Name(w323) -> ("total number of samples/ch"=w322:u32, "sound format"=w320:T2, "data"=w313:waveform(dbl)[])
            n245 = Divide(x=w303, y=100.0) -> (x/y=w307:dbl)
            n246 = Multiply(x=w304, y=w307) -> (x*y=w306:dbl)
            n247 = call <vilib>:"Sound Output Configure.vi"("number of samples/ch"=w322, "sample mode"=w321, "sound format"=w320, "device ID"=u32 0) -> ("error out"=w318:errorcluster, "task ID"=w319:T20)  [unwired: 6 in]
            n248 = call-poly <vilib>:"Sound Output Set Volume.vi"("error in (no error)"=w318, "volume"=w306, "task ID"=w319) -> ("error out"=w316:errorcluster, "task ID out"=w317:T20)  [unwired: 7 in]
            n249 = call <vilib>:"Sound Output Start.vi"("error in (no error)"=w316, "task ID"=w317) -> ("error out"=w314:errorcluster, "task ID out"=w315:T20)  [unwired: 8 in]
            n250 = call-poly <vilib>:"Sound Output Write.vi"("error in (no error)"=w314, "data"=w313, "task ID"=w315) -> ("error out"=w311:errorcluster, "task ID out"=w312:T20)  [unwired: 7 in]
            n251 = while {
              tunnel: w312 -> [w332]
              tunnel: w311 -> [w331]
              tunnel: [w330] -> w310
              tunnel: [w329] -> w309
              stop <- w324 continue-if-true
              n252 = call <vilib>:"Sound Output Info.vi"("error in (no error)"=w331, "task ID"=w332) -> ("error out"=w329:errorcluster, "is playing?"=w328:bool, "task ID out"=w330:T20)  [unwired: 6 in, 1 out]
              n253 = local read "Sound To Play"() -> (w326:T3)
              n254 = Equal?(x=w326, y=enum16{"None", "Start", "Stop", "Uh-Oh"}."None") -> (x = y?=w327:bool)
              n255 = And(x=w328, y=w327) -> (x .and. y?=w324:bool)
            }
            n256 = call <vilib>:"Sound Output Stop.vi"("error in (no error)"=w309, "task ID"=w310) -> ()  [unwired: 8 in, 2 out]
          }
        }
      }
    }
    n257 = local read "stop"() -> (w295:bool)
  }
